vi "Enqueue Message.vi"(8 "error in (no error)":errorcluster, 9 "Message Data":variant, 10 "Message":string, 11 "Process In":refnum<class "Debug Process.lvclass">) -> (0 "error out":errorcluster, 3 "Process Out":refnum<class "Debug Process.lvclass">)   [LabVIEW 2020, in "Debug Process.lvclass"]
uses:
  Debug Process.lvclass
  Debug Process.lvclass/Debug Process.ctl
  Message Cluster.ctl
  Request Message Cluster.ctl
  <vilib>/Utility/error.llb/Clear Errors.vi
  <vilib>/Utility/error.llb/Error Cluster From Error Code.vi
  <vilib>/ErrorRing/Error Ring.xnode
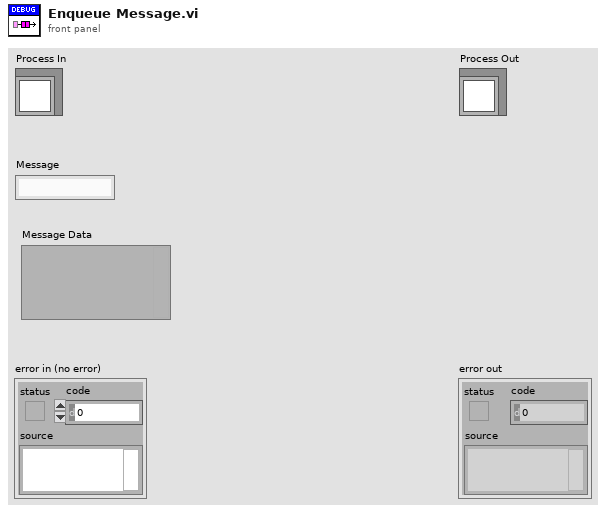
[diagram p1: front panel]
types:
  T1 = typedef "Debug Process.lvclass/Message Cluster.ctl" = cluster{"Message":string, "Message Data":variant, "Request Notifier":refnum<notifier>}
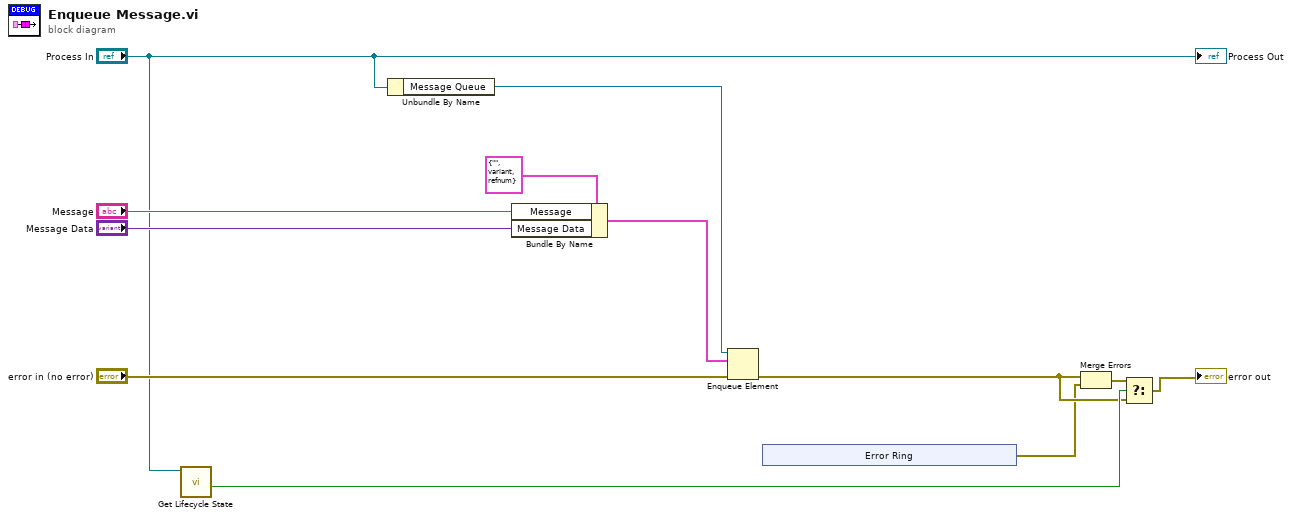
[diagram p0: block diagram]
diagram:
  n1 = call "Get Lifecycle State.vi"("Process In"="Process In") -> ("In Process Loop?"=w7:bool)  [unwired: 7 in, 3 out]
  n2 = Unbundle By Name("Process In") -> ("Message Queue"=w3:refnum<queue>)
  n3 = Bundle By Name(cluster=T1 {"Message"="", "Message Data"=variant, "Request Notifier"=refnum} ("Message Cluster"), "Message"="Message", "Message Data"="Message Data") -> (w2:T1)
  n4 = Enqueue Element(queue=w3, element=w2, error in (no error)="error in (no error)") -> (error out=w6:errorcluster)  [unwired: 1 in, 2 out]
  n5 = xnode "Error Ring"() -> ("error out"=w4:errorcluster)
  n6 = Merge Errors(w6, w4) -> (w5:errorcluster)
  n7 = Select(t=w5, s=w7, f=w6) -> (s? t:f=→"error out":errorcluster)
  "Process Out" <- "Process In"
